vi "子VI-修改评定结果.vi"(9 "全部检测结果":string[][](table), 11 "临界面积百分比值":dbl) -> (1 "全部检测结果合并输出":string[][](table) caption="全部检测结果")   [LabVIEW 2018]
panel:
  in  "ok":bool
  in  "确定按钮":bool
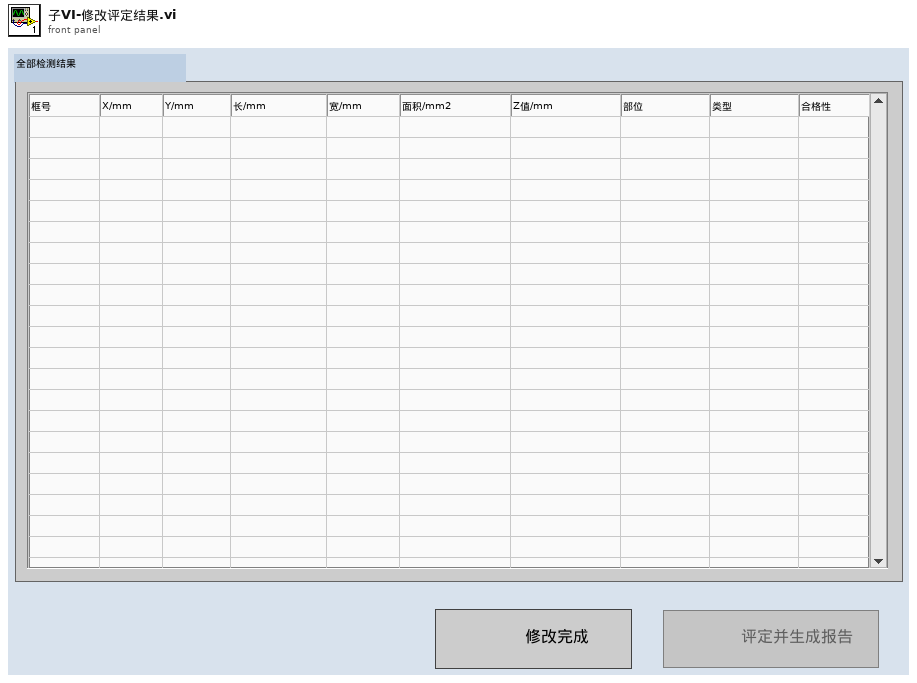
[diagram p1: front panel]
types:
  T1 = enum8{"Enabled", "Disabled", "Disabled and Grayed Out"}
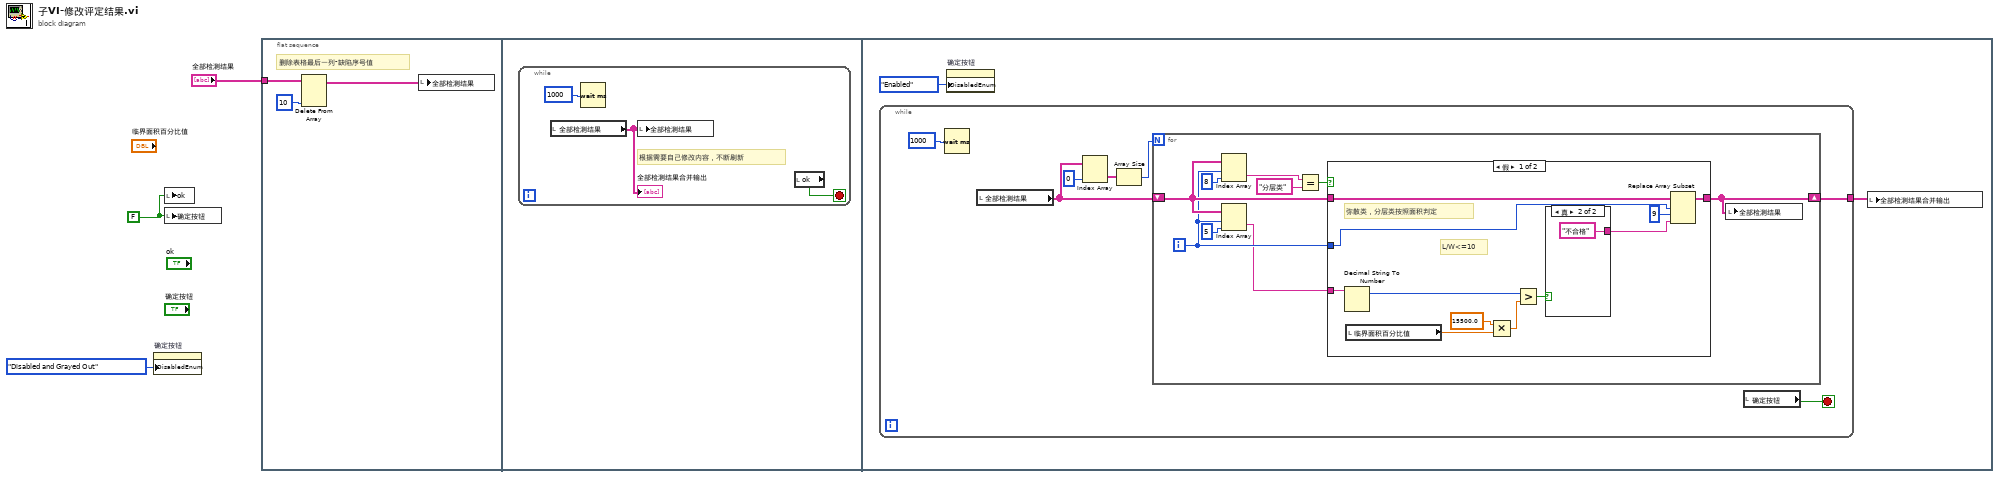
[diagram p0: block diagram]
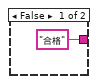
[diagram p2: hidden frame]
diagram:
  w3 = FALSE
  n1 = property on="确定按钮" class="Bool (严格)"("DisabledEnum"=T1."Disabled and Grayed Out" ("禁用")) -> ()  [unwired: 2 in, 2 out]
  n2 = local write "ok"(w3) -> ()
  n3 = local write "确定按钮"(w3) -> ()
  n4 = flat-sequence {
    tunnel: "全部检测结果" -> [w6]
    frame #0 {
      # "删除表格最后一列-缺陷序号值"
      n5 = Delete From Array(array=w6, index (col)=10 ("禁用的索引 (列)")) -> (array with subset deleted=w5:string[][])  [unwired: 2 in, 1 out]
      n6 = local write "全部检测结果"(w5) -> ()
    }
    frame #1 {
      n7 = while {
        stop <- w7 stop-if-true
        # "根据需要自己修改内容，不断刷新"
        n8 = local read "全部检测结果"() -> (w8:string[][])
        "全部检测结果合并输出" <- w8
        n9 = Wait (ms)(milliseconds to wait=u32 1000 ("等待时间（毫秒）")) -> ()  [unwired: 1 out]
        n10 = local write "全部检测结果"(w8) -> ()
        n11 = local read "ok"() -> (w7:bool)
      }
    }
    frame #2 {
      n12 = while {
        tunnel: [w13] -> w10
        stop <- w17 stop-if-true
        n13 = Wait (ms)(milliseconds to wait=u32 1000 ("等待时间（毫秒）")) -> ()  [unwired: 1 out]
        n14 = local read "全部检测结果"() -> (w14:string[][])
        n15 = Index Array(array=w14, index (col)=0 ("禁用的索引 (列)")) -> (element=w15:string[])  [unwired: 1 in]
        n16 = Array Size(array=w15) -> (size(s)=w18:i32)
        n17 = for {
          N: w18 -> [_]
          shift-right: [w19] -> w13
          shift-left: w14 -> [w23]
          i -> [w22]
          n18 = Index Array(array=w23, index (row)=w22, index (col)=8 ("禁用的索引 (列)")) -> (element=w25:string)
          n19 = Index Array(array=w23, index (row)=w22, index (col)=5 ("禁用的索引 (列)")) -> (element=w20:string)
          n20 = Equal?(x=w25, y="分层类") -> (x = y?=w24:bool)
          n21 = case shown="假" w24 {
            tunnel: w23 -> [w35 w41]
            tunnel: w22 -> [w34 _]
            tunnel: [w31 w41] -> w19
            tunnel: w20 -> [w29 _]
            frame False {
              # "L/W<=10"
              # "弥散类，分层类按照面积判定"
              n22 = Decimal String To Number(string=w29) -> (offset past number=w28:i32)  [unwired: 2 in, 1 out]
              n23 = local read "临界面积百分比值"() -> (w36:dbl)
              n24 = Multiply(x=15500.0, y=w36) -> (x*y=w38:dbl)
              n25 = Greater?(x=w28, y=w38) -> (0:w30:bool)
              n26 = case shown="真" w30 {
                tunnel: ["合格" "不合格"] -> w32
                frame False {
                }
                frame True {
                }
              }
              n27 = Replace Array Subset(array=w35, new element=w32, index (row)=w34, index (col)=9 ("禁用的索引 (列)")) -> (w31:string[][])
            }
            frame True {
              # "分层类，合格性按照Z值\n默认不变"
            }
          }
          n28 = local write "全部检测结果"(w19) -> ()
        }
        n29 = local read "确定按钮"() -> (w17:bool)
      }
      n30 = property on="确定按钮" class="Bool (严格)"("DisabledEnum"=T1."Enabled" ("禁用")) -> ()  [unwired: 2 in, 2 out]
      n31 = local write "全部检测结果合并输出"(w10) -> ()
    }
  }
